vi "DisplayErrorsToUser.vi"() -> ()   [LabVIEW 2011]
panel:
  out "Current Number of Errors:\nOnly Returns the Last 100":i32
  in  "Cancel Button":bool
  out "Error source":string[](array[string])
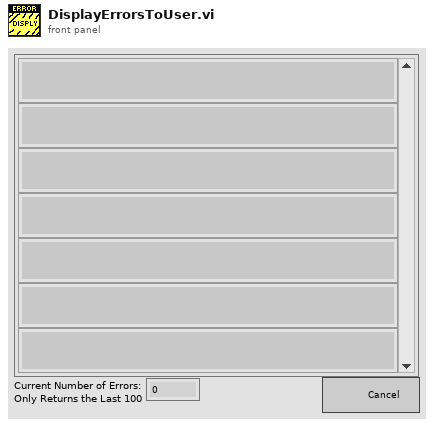
[diagram p1: front panel]
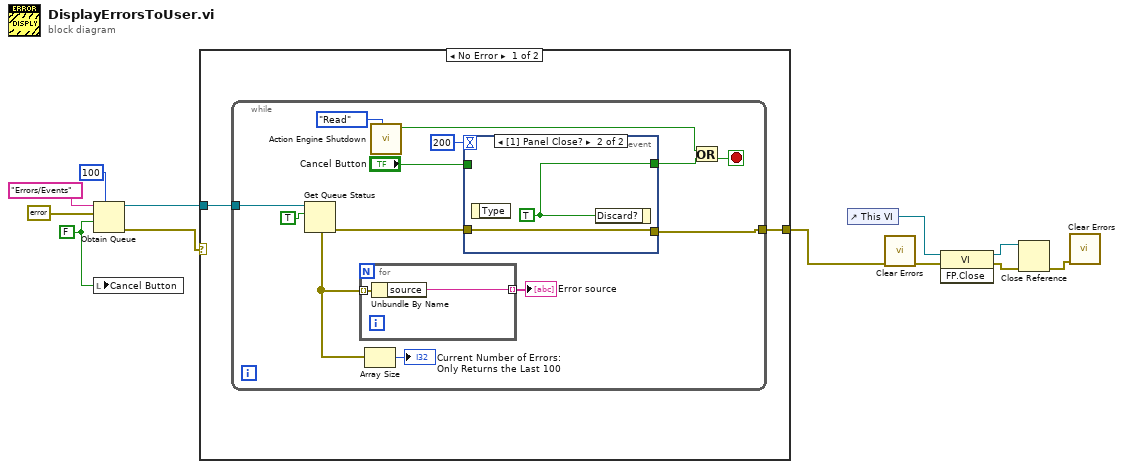
[diagram p0: block diagram]
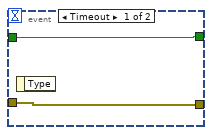
[diagram p2: hidden frame]
diagram:
  w4 = FALSE ("create if not found? (T)")
  n1 = Obtain Queue(max queue size (-1, unlimited)=100, name (unnamed)="Errors/Events", element data type=errorcluster {"status"=FALSE, "code"=0, "source"=""} ("error constant"), create if not found? (T)=w4) -> (queue out=w10:refnum<queue>, error out=w8:errorcluster)  [unwired: 1 in, 1 out]
  n2 = local write "Cancel Button"(w4) -> ()
  n3 = case shown="No Error" w8 {
    selector: w8 -> [_ w34]
    tunnel: w10 -> [w14 _]
    tunnel: [w13 w34] -> w5
    frame No Error {
      n4 = while {
        tunnel: w14 -> [w27]
        tunnel: [w18] -> w13
        stop <- w21 stop-if-true
        n5 = Get Queue Status(queue=w27, return elements? (F)=TRUE) -> (error out=w19:errorcluster, elements=w24:errorcluster[])  [unwired: 1 in, 6 out]
        n6 = for {
          tunnel: w24 -> [w33] mode=indexing
          tunnel: [w32] -> w25 mode=indexing
          n7 = Unbundle By Name(w33) -> ("source"=w32:string)
        }
        "Error source" <- w25
        n8 = Array Size(array=w24) -> (size(s)=→"Current Number of Errors:\nOnly Returns the Last 100":i32)
        n9 = call "Action Engine Shutdown.vi"("Shutdown"=enum16{"Write", "Read"}."Read") -> ("Shutdown"=w20:bool)  [unwired: 9 in, 1 out]
        n10 = event shown="[1] Panel Close?" {
          selector: _ -> [_ _]
          dyn-events: _ -> [_ _]
          timeout: 200 -> [_ _]
          tunnel: w19 -> [w29 w31]
          tunnel: [w29 w31] -> w18
          tunnel: "Cancel Button" -> [w28 _]
          tunnel: [w28 w30] -> w15
          event Timeout {
            n11 = event-data() -> ()  [unwired: 1 in, 1 out]
          }
          event Panel Close? {
            w30 = TRUE ("Discard?")
            n12 = event-data() -> ()  [unwired: 1 in, 1 out]
            n13 = event-data("Discard?"=w30) -> ()  [unwired: 1 in, 1 out]
          }
        }
        n14 = Or(x=w20, y=w15) -> (x .or. y?=w21:bool)
      }
    }
    frame Error {
    }
  }
  n15 = control-ref of="This VI"() -> (w7:refnum<vi>)
  n16 = call <vilib>:"Clear Errors.vi"("error in (no error)"=w5) -> ("error out"=w6:errorcluster)  [unwired: 6 in]
  n17 = invoke class="VI" method="FP.Close"(reference=w7, error in=w6) -> (reference out=w2:refnum<vi>, error out=w3:errorcluster)  [unwired: 1 in, 1 out]
  n18 = Close Reference(reference=w2, error in (no error)=w3) -> (error out=w1:errorcluster)
  n19 = call <vilib>:"Clear Errors.vi"("error in (no error)"=w1) -> ()  [unwired: 6 in, 1 out]
